vi "TestGetBrightness.vi"() -> ()   [LabVIEW 2019]
panel:
  in  "Exposure (us)":u32
  out "brightness":dbl
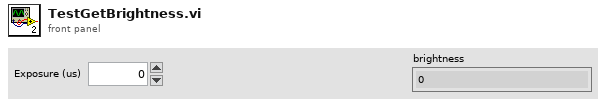
[diagram p1: front panel]
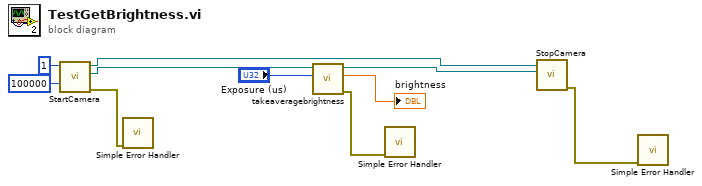
[diagram p0: block diagram]
diagram:
  n1 = call "StartCamera.vi"("ExposureTime_us"=u32 100000, "Gain"=u32 1) -> ("Error Out"=w8:errorcluster, "TLCamera reference out"=w6:refnum<k24>, "TLCameraSDK reference out"=w5:refnum<k24>)  [unwired: 7 in]
  n2 = call <vilib>:"Simple Error Handler.vi"("error in (no error)"=w8) -> ()  [unwired: 4 in, 5 out]
  n3 = call "takeaveragebrightness.vi"("Exposure (us)"="Exposure (us)", "TLCamera reference in"=w6) -> ("Error Out"=w2:errorcluster, "brightness"=→"brightness":dbl, "TLCamera reference out"=w4:refnum<k24>)  [unwired: 7 in]
  n4 = call <vilib>:"Simple Error Handler.vi"("error in (no error)"=w2) -> ()  [unwired: 4 in, 5 out]
  n5 = call "StopCamera.vi"("TLCamera reference"=w4, "TLCameraSDK reference"=w5) -> ("Error Out"=w7:errorcluster)  [unwired: 9 in]
  n6 = call <vilib>:"Simple Error Handler.vi"("error in (no error)"=w7) -> ()  [unwired: 4 in, 5 out]
